vi "Read Attributes.vi"(11 "Set DER VF Msg":refnum<class "Set DER VF Msg.lvclass">) -> (2 "Payload":cluster{"DER_VF":T1})   [LabVIEW 2018, in "Device Communication and Control Abstract Actor.lvlib" / "Set DER VF Msg.lvclass"]
uses:
  Set DER VF Msg.lvclass
  <vilib>/ORNL/CSEISMIC DDS/CSEISMIC DDS Base/Data Types/DER_VF.ctl
  <vilib>/ORNL/CSEISMIC DDS/CSEISMIC DDS Base/Data Types/Controls/DeviceID.ctl
  Set DER VF Msg.lvclass/Set DER VF Msg.ctl
  <vilib>/ORNL/CSEISMIC DDS/CSEISMIC DDS Base/CSEISMIC DDS.lvclass
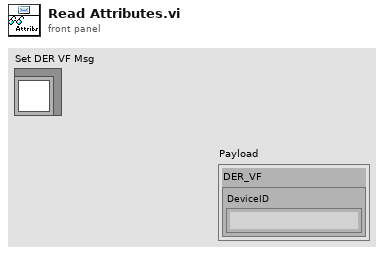
[diagram p1: front panel]
types:
  T1 = typedef "CSEISMIC DDS.lvlib/CSEISMIC DDS.lvclass/DER_VF.ctl" = cluster{"DeviceID":T2}
  T2 = typedef "CSEISMIC DDS.lvlib/CSEISMIC DDS.lvclass/DeviceID.ctl" = string
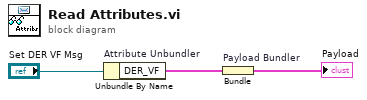
[diagram p0: block diagram]
diagram:
  n1 = Unbundle By Name "Attribute Unbundler"("Set DER VF Msg") -> ("DER_VF"=w1:T1)
  n2 = Bundle "Payload Bundler"("DER_VF"=w1) -> (→"Payload":cluster{"DER_VF":T1})  [unwired: 1 in]
